vi "Wrapper_ClosePicture+File.vi"(8 "error in (no error)":errorcluster, 10 "LIMPICTURE":T2, 11 "hFile in":T1) -> (0 "error out":errorcluster)   [LabVIEW 2014, in "ND2_Reader_32.lvlib"]
uses:
  ND2_Reader_32.lvlib
  controls/cluster_LIMPICTURE.ctl
  controls/numeric_LIMFILEHANDLE.ctl
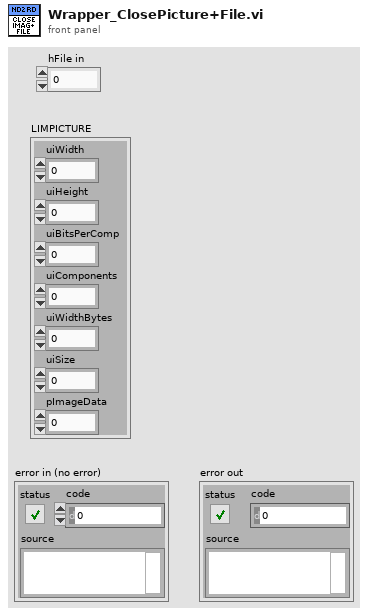
[diagram p1: front panel]
types:
  T1 = typedef "numeric_LIMFILEHANDLE.ctl" = i32
  T2 = typedef "cluster_LIMPICTURE.ctl" = cluster{"uiWidth":u32, "uiHeight":u32, "uiBitsPerComp":u32, "uiComponents":u32, "uiWidthBytes":u32, "uiSize":u32, "pImageData":u32}
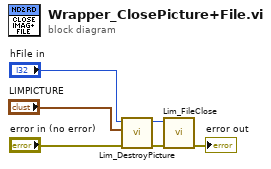
[diagram p0: block diagram]
diagram:
  n1 = call "Lim_DestroyPicture.vi"("error in (no error)"="error in (no error)", "LIMPICTURE"="LIMPICTURE", "hFile in"="hFile in") -> ("error out"=w1:errorcluster, "hFile out"=w2:T1)  [unwired: 7 in]
  n2 = call "Lim_FileClose.vi"("error in (no error)"=w1, "hFile in"=w2) -> ("error out"=→"error out":errorcluster)  [unwired: 8 in, 1 out]
